vi "closeInterface.vi"(8 "error in (no error)":errorcluster, 10 "interface object in":refnum<k20>, 11 "Orion_BMS in":refnum<class "Orion_BMS.lvclass">) -> (0 "error out":errorcluster, 3 "Orion_BMS out":refnum<class "Orion_BMS.lvclass">)   [LabVIEW 2017, in "Orion_BMS.lvclass"]
uses:
  Orion_BMS.lvclass
  <vilib>/CANopenLib/CANOPEN.llb/CANopen Interface Close.vi
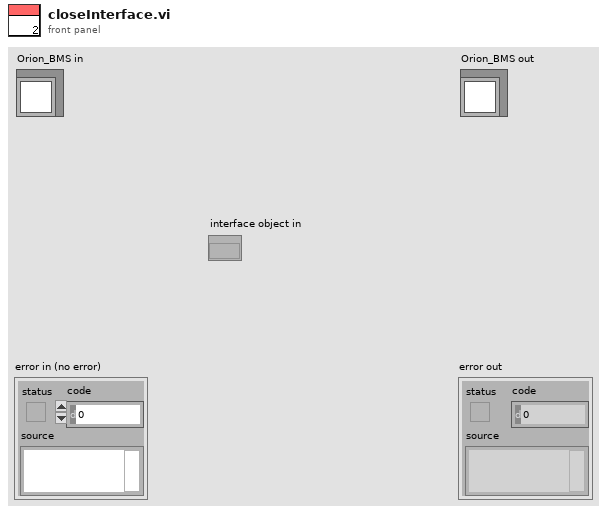
[diagram p1: front panel]
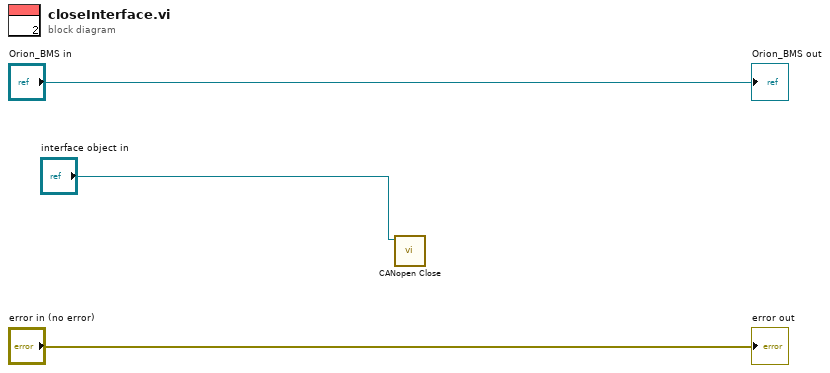
[diagram p0: block diagram]
diagram:
  n1 = call-poly <vilib>:"CANopen Close.vi"("interface object in"="interface object in") -> ()  [unwired: 10 in, 1 out]
  "error out" <- "error in (no error)"
  "Orion_BMS out" <- "Orion_BMS in"
